vi "Determine Transmit.vi"(7 "Current Time":u32, 9 "Detect?":bool[](array[boolean]), 10 "Values":dbl[](array[numeric]), 11 "Frame Settings in":T1 {"Protection Configurations"."CRC Channels"."Data Type" items=["Signed", "Unsigned", "IEEE Float"]}) -> (1 "Transmit":bool, 2 "Values out":dbl[](array[numeric]), 3 "Frame Settings out":T1 {"Protection Configurations"."CRC Channels"."Data Type" items=["Signed", "Unsigned", "IEEE Float"]})   [LabVIEW 2023, in "Protection and Counter Support Engine.lvlib"]
uses:
  Protection and Counter Support Engine.lvlib
  Types/RT Frame Settings.ctl
  Shared/Types/Exported Frame Type.ctl
  Types/RT Protection Configuration.ctl
  Shared/Types/Protection Type.ctl
  Shared/Types/XNET Signal Configuration.ctl
  Shared/Types/Exported Counter Settings.ctl
  Shared/Types/Exported Event Trigger Type.ctl
  Shared/Protection and Counter Support Shared.lvlib
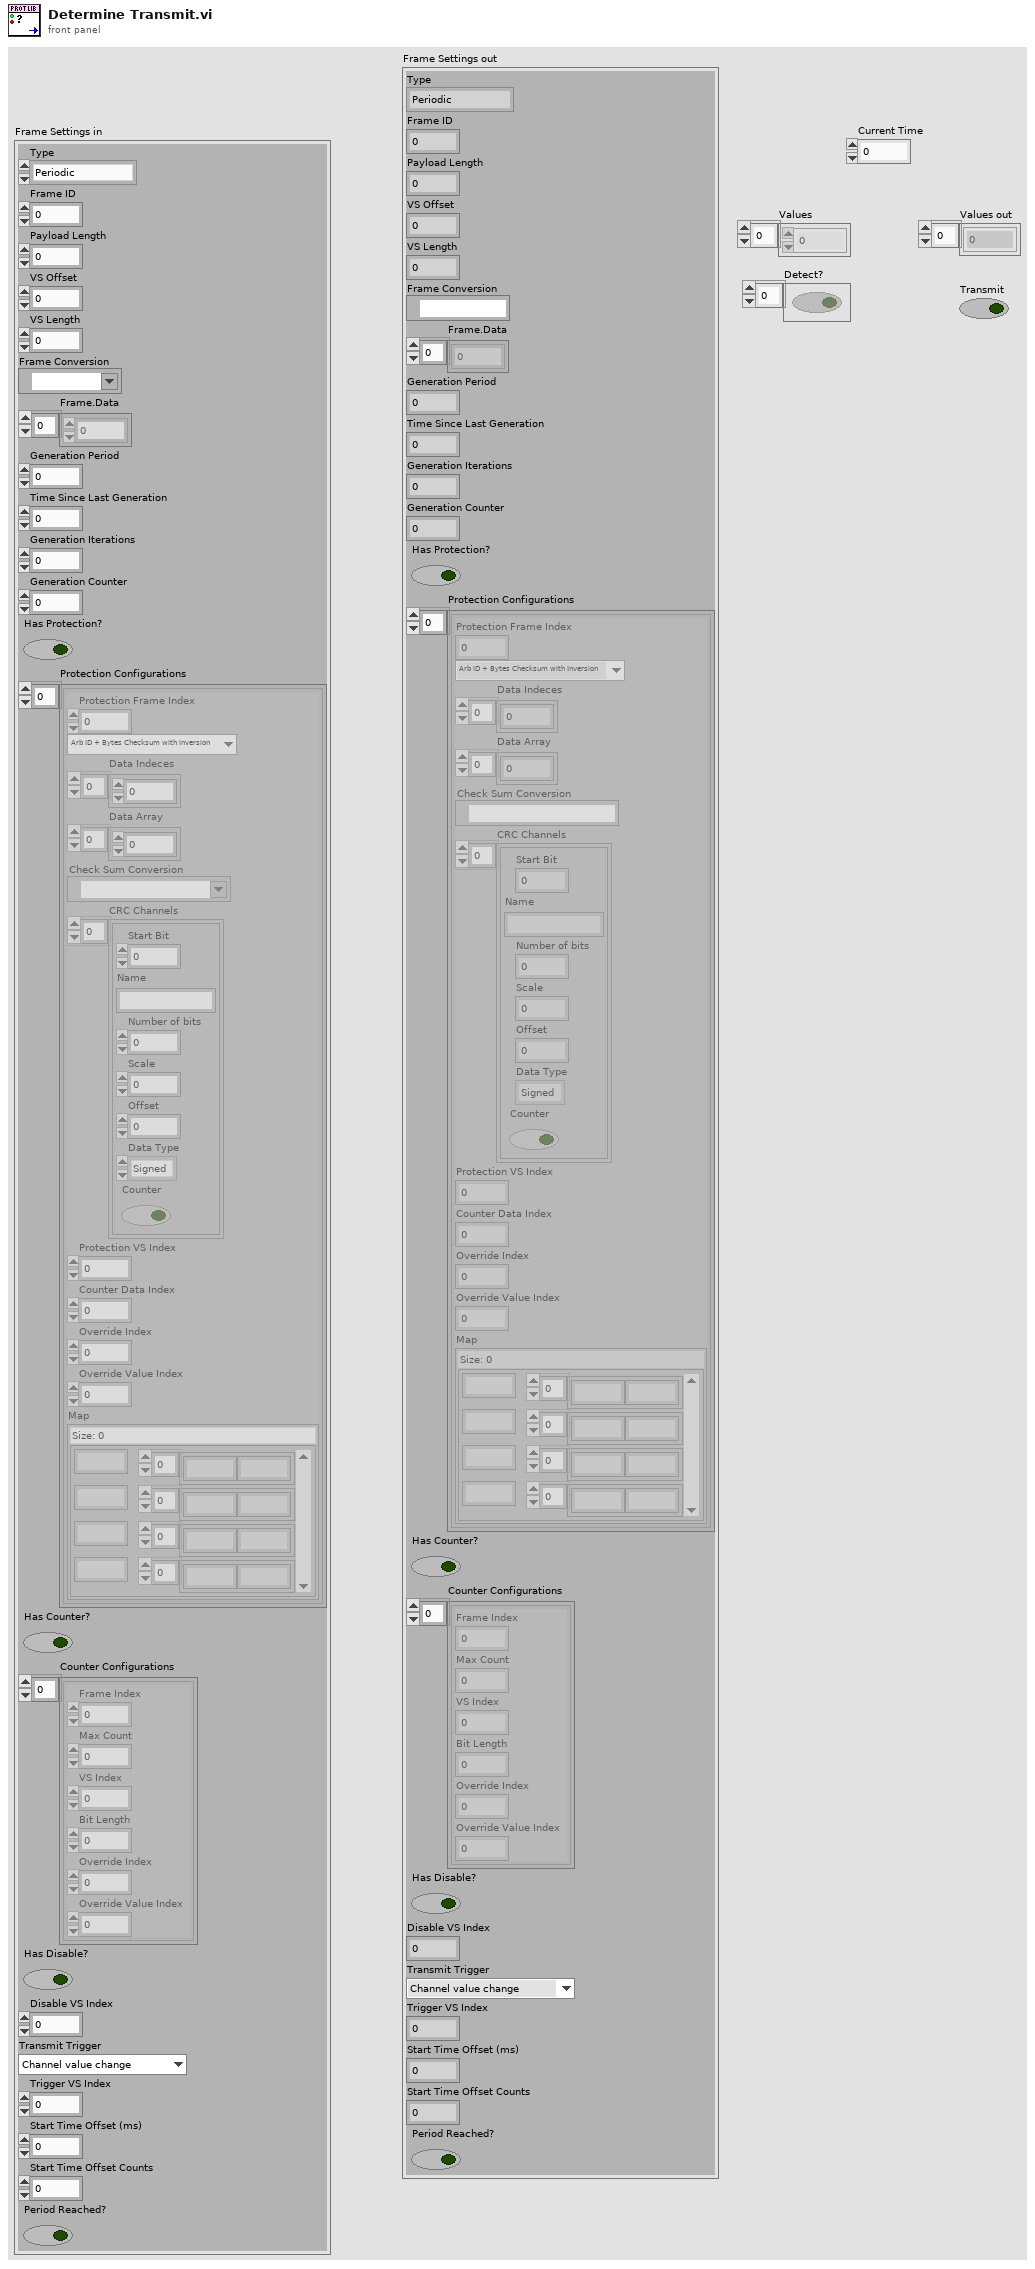
[diagram p1: front panel]
types:
  T1 = typedef "Protection and Counter Support Engine.lvlib/RT Frame Settings.ctl" = cluster{"Type":T2, "Frame ID":u32, "Payload Length":u32, "VS Offset":i32, "VS Length":i32, "Frame Conversion":refnum<k21>, "Frame.Data":dbl[], "Generation Period":u32, "Time Since Last Generation":u32, "Generation Iterations":u32, "Generation Counter":u32, "Has Protection?":bool, "Protection Configurations":T3[], "Has Counter?":bool, "Counter Configurations":T6[], "Has Disable?":bool, "Disable VS Index":i32, "Transmit Trigger":T7, "Trigger VS Index":i32, "Start Time Offset (ms)":u32, "Start Time Offset Counts":u32, "Period Reached?":bool}
  T2 = typedef "Protection and Counter Support Shared.lvlib/Exported Frame Type.ctl" = enum16{"Periodic", "Event", "Periodic/Event"}
  T3 = typedef "Protection and Counter Support Engine.lvlib/RT Protection Configuration.ctl" = cluster{"Protection Frame Index":i32, "Protection Type":T4, "Data Indeces":i32[], "Data Array":dbl[], "Check Sum Conversion":refnum<k21>, "CRC Channels":T5[], "Protection VS Index":i32, "Counter Data Index":i32, "Override Index":i32, "Override Value Index":i32, "Map":map{i32, u8[]}}
  T4 = typedef "Protection and Counter Support Shared.lvlib/Protection Type.ctl" = enum16{"Arb ID + Bytes Checksum with Inversion", "Arb ID + Bytes CRC with Inversion", "Reversed Raw Signal Checksum with Inversion", "Concatenated Two's Compliment", "LP_CRC8", "LP_Checksum", "LP_CRC8_MRS"}
  T5 = typedef "Protection and Counter Support Shared.lvlib/XNET Signal Configuration.ctl" = cluster{"Start Bit":i32, "Name":string, "Number of bits":i32, "Scale":dbl, "Offset":dbl, "Data Type":u32, "Counter":bool}
  T6 = typedef "Protection and Counter Support Shared.lvlib/Exported Counter Settings.ctl" = cluster{"Frame Index":i32, "Max Count":dbl, "VS Index":i32, "Bit Length":i64, "Override Index":i32, "Override Value Index":i32}
  T7 = typedef "Protection and Counter Support Shared.lvlib/Exported Event Trigger Type.ctl" = enum16{"Channel value change", "Trigger channel (not zero)", "Channel value change or trigger channel (not zero)", "Trigger channel (any value change)", "Channel value change or trigger channel (any value change)"}
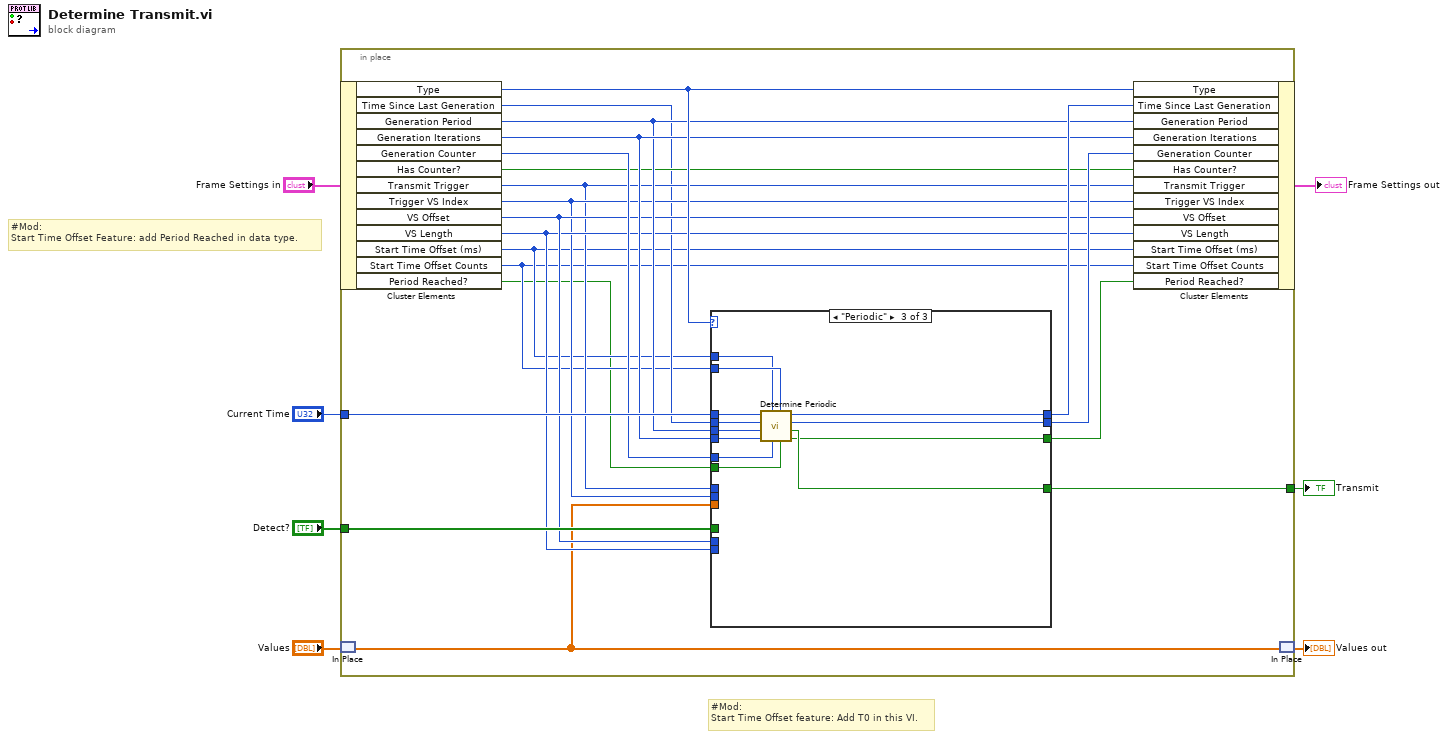
[diagram p0: block diagram]
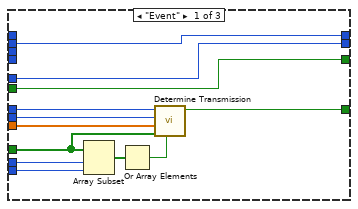
[diagram p2: hidden frame]
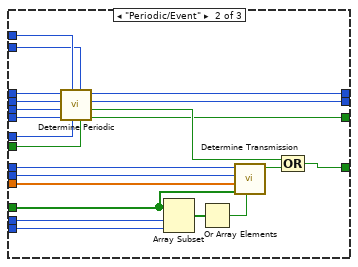
[diagram p3: hidden frame]
diagram:
  # "#Mod:\nStart Time Offset Feature: add Period Reached in data type."
  # "#Mod:\nStart Time Offset feature: Add T0 in this VI."
  n1 = in-place {
    in-place-border: [w27] -> w7
    in-place-border: "Detect?" -> [w26]
    in-place-border: "Current Time" -> [w25]
    n2 = in-place-cluster #1("Frame Settings in") -> ("Type"=w23:T2, "Time Since Last Generation"=w12:u32, "Generation Period"=w19:u32, "Generation Iterations"=w20:u32, "Generation Counter"=w24:u32, "Has Counter?"=w18:bool, "Transmit Trigger"=w14:T7, "Trigger VS Index"=w15:i32, "VS Offset"=w17:i32, "VS Length"=w16:i32, "Start Time Offset (ms)"=w11:u32, "Start Time Offset Counts"=w10:u32, "Period Reached?"=w9:bool)
    n3 = in-place-match #2("Values") -> (w13:dbl[])
    n4 = case shown="\"Periodic\"" w23 {
      tunnel: w19 -> [_ w51 w73]
      tunnel: w12 -> [w39 w50 w72]
      tunnel: w25 -> [_ w49 w71]
      tunnel: [w39 w48 w70] -> w22
      tunnel: w24 -> [w38 w53 w66]
      tunnel: w20 -> [_ w52 w67]
      tunnel: [w31 w44 w69] -> w27
      tunnel: [w38 w47 w68] -> w21
      tunnel: w14 -> [w33 w57 _]
      tunnel: w15 -> [w34 w58 _]
      tunnel: w16 -> [w37 w61 _]
      tunnel: w17 -> [w36 w60 _]
      tunnel: w26 -> [w30 w55 _]
      tunnel: w13 -> [w29 w54 _]
      tunnel: w11 -> [_ w43 w62]
      tunnel: w10 -> [_ w42 w63]
      tunnel: w9 -> [w28 w41 w64]
      tunnel: [w28 w40 w65] -> w8
      frame "Event" {
        n5 = Array Subset(array=w30, index=w36, length=w37) -> (w35:bool[])
        n6 = Or Array Elements(Boolean array=w35) -> (logical OR=w32:bool)
        n7 = call "Determine Transmission.vi"("Channel Value Change"=w32, "Detect?"=w30, "Values"=w29, "Trigger VS Index"=w34, "Transmit Trigger"=w33) -> ("Transmit"=w31:bool)  [unwired: 6 in]
      }
      frame "Periodic/Event" {
        n8 = call "Determine Periodic.vi"("Period Reached?"=w41, "Start Time Offset Counts"=w42, "Generation Counter"=w53, "Start Time Offset"=w43, "Generation Iterations"=w52, "Generation Period"=w51, "Time Since Last Generation in"=w50, "Current Time"=w49) -> ("Period Reached out"=w40:bool, "Transmit"=w46:bool, "Generation Counter out"=w47:u32, "Time Since Last Generation out"=w48:u32)
        n9 = Array Subset(array=w55, index=w60, length=w61) -> (w59:bool[])
        n10 = Or Array Elements(Boolean array=w59) -> (logical OR=w56:bool)
        n11 = call "Determine Transmission.vi"("Channel Value Change"=w56, "Detect?"=w55, "Values"=w54, "Trigger VS Index"=w58, "Transmit Trigger"=w57) -> ("Transmit"=w45:bool)  [unwired: 6 in]
        n12 = Compound Arithmetic op=OR(w46, w45) -> (w44:bool)
      }
      frame "Periodic" {
        n13 = call "Determine Periodic.vi"("Period Reached?"=w64, "Start Time Offset Counts"=w63, "Generation Counter"=w66, "Start Time Offset"=w62, "Generation Iterations"=w67, "Generation Period"=w73, "Time Since Last Generation in"=w72, "Current Time"=w71) -> ("Period Reached out"=w65:bool, "Transmit"=w69:bool, "Generation Counter out"=w68:u32, "Time Since Last Generation out"=w70:u32)
      }
    }
    n14 = in-place-cluster #1("Type"=w23, "Time Since Last Generation"=w22, "Generation Period"=w19, "Generation Iterations"=w20, "Generation Counter"=w21, "Has Counter?"=w18, "Transmit Trigger"=w14, "Trigger VS Index"=w15, "VS Offset"=w17, "VS Length"=w16, "Start Time Offset (ms)"=w11, "Start Time Offset Counts"=w10, "Period Reached?"=w8) -> (→"Frame Settings out":T1)
    n15 = in-place-match #2(w13) -> (→"Values out":dbl[])
  }
  "Transmit" <- w7
